vi "sub_est_noise_power - MS.vi"(8 "Bin Size":i32=100, 10 "Input Complex Samples":cdb[](array[numeric])) -> (0 "Energy Threshold":dbl, 2 "noise_power":dbl, 4 "signal_power":dbl, 5 "noise_estimation_error ?":bool)   [LabVIEW 2010]
uses:
  <vilib>/imath/engines/lvmath2/RunTimeEngine/BuiltInFunctions/max/2 inputs/NIMS_max(RG,RG)-no size check.vi
  <instcachedir>/0/NIMS_max(RG,RG)-no size check_F871939977644B7683C1350DCCAD7557.lvgen/NIMS_max(RG,RG)-no size check_F871939977644B7683C1350DCCAD7557_001.vi
  <vilib>/imath/engines/lvmath2/RunTimeEngine/BuiltInFunctions/min/1 input/NIMS_min(RV).vi
  <instcachedir>/0/NIMS_min(RV)_EE2DD3E2888846108C5160A664B67832.lvgen/NIMS_min(RV)_EE2DD3E2888846108C5160A664B67832_000.vi
  <vilib>/imath/engines/lvmath2/RunTimeEngine/BuiltInFunctions/max/1 input/NIMS_max(RV).vi
  <instcachedir>/0/NIMS_max(RV)_237633DB1D604D5BA7001287DF3C7957.lvgen/NIMS_max(RV)_237633DB1D604D5BA7001287DF3C7957_000.vi
  <vilib>/imath/engines/lvmath2/RunTimeEngine/NodeEndStatement/NIMS_NodeEndStatement_Output.vi
  <instcachedir>/0/NIMS_NodeEndStatement_Output_53EC0D466D134D7ABD903AC30B43404B.lvgen/NIMS_NodeEndStatement_Output_53EC0D466D134D7ABD903AC30B43404B_001.vi
  <instcachedir>/0/NIMS_NodeEndStatement_Output_53EC0D466D134D7ABD903AC30B43404B.lvgen/NIMS_NodeEndStatement_Output_53EC0D466D134D7ABD903AC30B43404B_010.vi
  <vilib>/imath/engines/lvmath2/RunTimeEngine/ErrorHandling/NIMS_Finalize Error.vi
panel:
  out "power":dbl[](array[numeric])
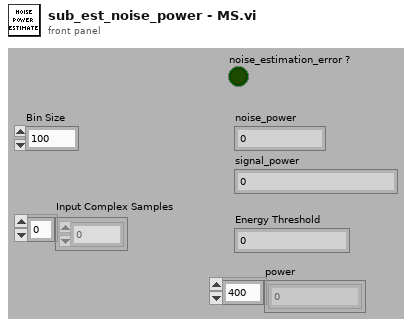
[diagram p1: front panel]
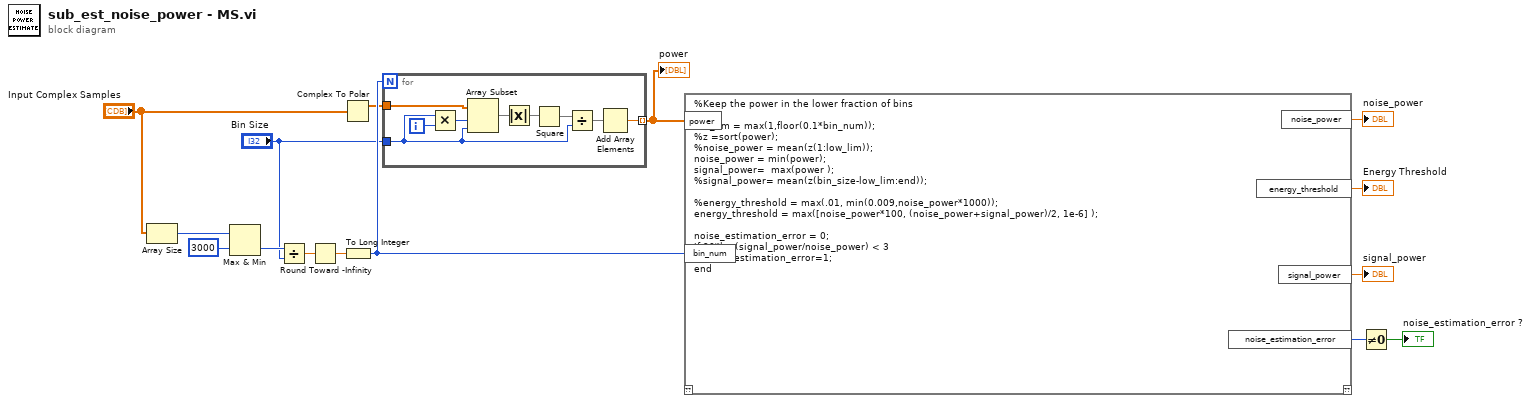
[diagram p0: block diagram]
diagram:
  n1 = Array Size(array="Input Complex Samples") -> (size(s)=w7:i32)
  n2 = Max & Min(x=w7, y=3000) -> (min(x,y)=w6:i32)  [unwired: 1 out]
  n3 = Divide(x=w6, y="Bin Size") -> (x/y=w10:dbl)
  n4 = Round Toward -Infinity(1:w10) -> (0:w9:dbl)
  n5 = Complex To Polar(r * e^(i*theta)="Input Complex Samples") -> (r=w2:dbl[])  [unwired: 1 out]
  n6 = To Long Integer(number=w9) -> (32bit integer=w4:i32)
  n7 = for {
    N: w4 -> [_]
    tunnel: w2 -> [w24]
    tunnel: "Bin Size" -> [w18]
    tunnel: [w19] -> w1 mode=indexing
    i -> [w17]
    n8 = Multiply(x=w18, y=w17) -> (x*y=w16:i32)
    n9 = Array Subset(array=w24, index=w16, length=w18) -> (w23:dbl[])
    n10 = Absolute Value(x=w23) -> (abs(x)=w22:dbl[])
    n11 = Square(x=w22) -> (x^2=w21:dbl[])
    n12 = Divide(x=w21, y=w18) -> (x/y=w20:dbl[])
    n13 = Add Array Elements(numeric array=w20) -> (sum=w19:dbl)
  }
  "power" <- w1
  n14 = mathscript code="%Keep the power in the lower fraction of bins\n\nlow_lim = max(1,floor(0.1*bin_num));\n%z =sort(power);\n%noise_power = mean(z(1:low_lim));  \nnoise_power = min(power);\nsignal_power=  max(power );\n%signal_power= mean(z(bin_size-low_lim:end)); \n\n%energy_threshold = max(.01, min(0.009,noise_power*1000));\nenergy_threshold = max([noise_power*100, (noise_power+signal_power)/2, 1e-6] );\n\nnoise_estimation_error = 0;\nif 20*log(signal_power/noise_power) < 3\n   noise_estimation_error=1;\nend"("power"=w1, "bin_num"=w4) -> ("noise_power"=→"noise_power":dbl, "signal_power"=→"signal_power":dbl, "energy_threshold"=→"Energy Threshold":dbl, "noise_estimation_error"=w12:i32)  [unwired: 1 in, 1 out]
  n15 = Not Equal To 0?(x=w12) -> (x != 0?=→"noise_estimation_error ?":bool)
